vi "stepper_motor_control.vi"() -> ()   [LabVIEW 2023]
panel:
  in  "Direction":string="1"
  in  "Steps":string="2000"
  in  "Speed":string="1000"
  out "error out":errorcluster
  in  "VISA resource name":refnum<visa-resource-name>
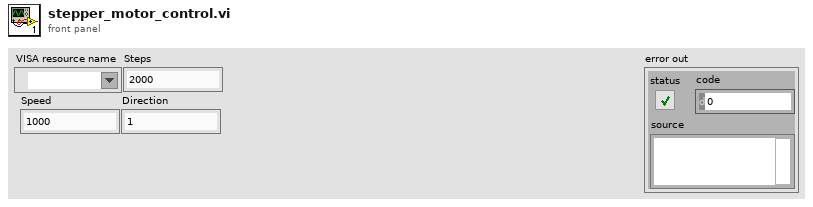
[diagram p1: front panel]
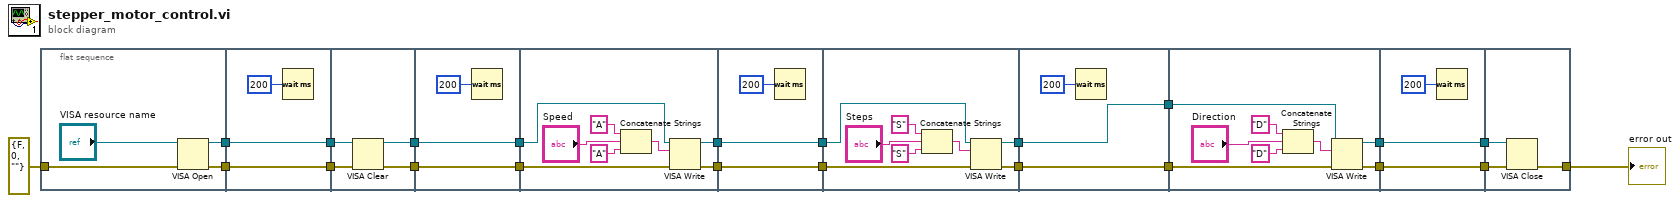
[diagram p0: block diagram]
diagram:
  n1 = flat-sequence {
    tunnel: [w25] -> w21
    tunnel: [w24] -> w13
    tunnel: errorcluster {"status"=FALSE, "code"=0, "source"=""} ("error in (no error)") -> [w23]
    tunnel: [w28] -> w17
    tunnel: w21 -> [w28]
    tunnel: [w27] -> w14
    tunnel: w13 -> [w27]
    tunnel: w17 -> [w33]
    tunnel: [w32] -> w16
    tunnel: w14 -> [w31]
    tunnel: [w30] -> w11
    tunnel: w16 -> [w36]
    tunnel: [w36] -> w15
    tunnel: [w34] -> w12
    tunnel: w11 -> [w34]
    tunnel: w15 -> [w44]
    tunnel: [w43] -> w19
    tunnel: w12 -> [w42]
    tunnel: [w41] -> w9
    tunnel: [w46] -> w20
    tunnel: w19 -> [w46]
    tunnel: [w45] -> w10
    tunnel: w9 -> [w45]
    tunnel: w20 -> [w55]
    tunnel: [w54] -> w18
    tunnel: w10 -> [w53]
    tunnel: [w52] -> w8
    tunnel: w18 -> [w56]
    tunnel: [w57] -> w4
    tunnel: w8 -> [w57]
    tunnel: [w56] -> w1
    tunnel: [w66] -> w22
    tunnel: [w65] -> w7
    tunnel: w4 -> [w60]
    tunnel: w1 -> [w59]
    tunnel: [w69] -> w3
    tunnel: [w68] -> w2
    tunnel: w7 -> [w68]
    tunnel: w22 -> [w69]
    tunnel: w3 -> [w72]
    tunnel: w2 -> [w71]
    tunnel: [w70] -> w6
    frame #0 {
      n2 = VISA Open(error in (no error)=w23, VISA resource name="VISA resource name") -> (VISA resource name=w25:refnum<visa-resource-name>, error out=w24:errorcluster)  [unwired: 3 in]
    }
    frame #1 {
      n3 = Wait (ms)(milliseconds to wait=u32 200) -> ()  [unwired: 1 out]
    }
    frame #2 {
      n4 = VISA Clear(VISA resource name=w33, error in (no error)=w31) -> (VISA resource name out=w32:refnum<visa-resource-name>, error out=w30:errorcluster)
    }
    frame #3 {
      n5 = Wait (ms)(milliseconds to wait=u32 200) -> ()  [unwired: 1 out]
    }
    frame #4 {
      n6 = Concatenate Strings("A" ("write buffer"), "Speed", "A" ("string")) -> (w37:string)
      n7 = VISA Write(VISA resource name=w44, write buffer=w37, error in (no error)=w42) -> (VISA resource name out=w43:refnum<visa-resource-name>, error out=w41:errorcluster)  [unwired: 1 out]
    }
    frame #5 {
      n8 = Wait (ms)(milliseconds to wait=u32 200) -> ()  [unwired: 1 out]
    }
    frame #6 {
      n9 = Concatenate Strings("S" ("write buffer"), "Steps", "S" ("string")) -> (w48:string)
      n10 = VISA Write(VISA resource name=w55, write buffer=w48, error in (no error)=w53) -> (VISA resource name out=w54:refnum<visa-resource-name>, error out=w52:errorcluster)  [unwired: 1 out]
    }
    frame #7 {
      n11 = Wait (ms)(milliseconds to wait=u32 200) -> ()  [unwired: 1 out]
    }
    frame #8 {
      n12 = Concatenate Strings("D" ("write buffer"), "Direction", "D" ("string")) -> (w62:string)
      n13 = VISA Write(VISA resource name=w59, write buffer=w62, error in (no error)=w60) -> (VISA resource name out=w66:refnum<visa-resource-name>, error out=w65:errorcluster)  [unwired: 1 out]
    }
    frame #9 {
      n14 = Wait (ms)(milliseconds to wait=u32 200) -> ()  [unwired: 1 out]
    }
    frame #10 {
      n15 = VISA Close(VISA resource name=w72, error in (no error)=w71) -> (error out=w70:errorcluster)
    }
  }
  "error out" <- w6
